vi "ConvertTextBasedCodeToLabVIEW_AttToHtml.vi"(7 "MissingClasses":string[](array[string]), 10 "ShowAccesScope(True)":bool=TRUE, 11 "DataType":T1) -> (3 "String":string)   [LabVIEW 2020]
uses:
  <resource>/Framework/Providers/Open_GDS/ClassProviders/Common/CommonVIs/CommonVIs_AttributeType.ctl
  <resource>/Framework/Providers/Open_GDS/ClassProviders/Common/CommonVIs/CommonVIs_AttributeDataType.ctl
  <resource>/Framework/Providers/Open_GDS/ClassProviders/Common/String/GDSString_AccessScopeModifierType.ctl
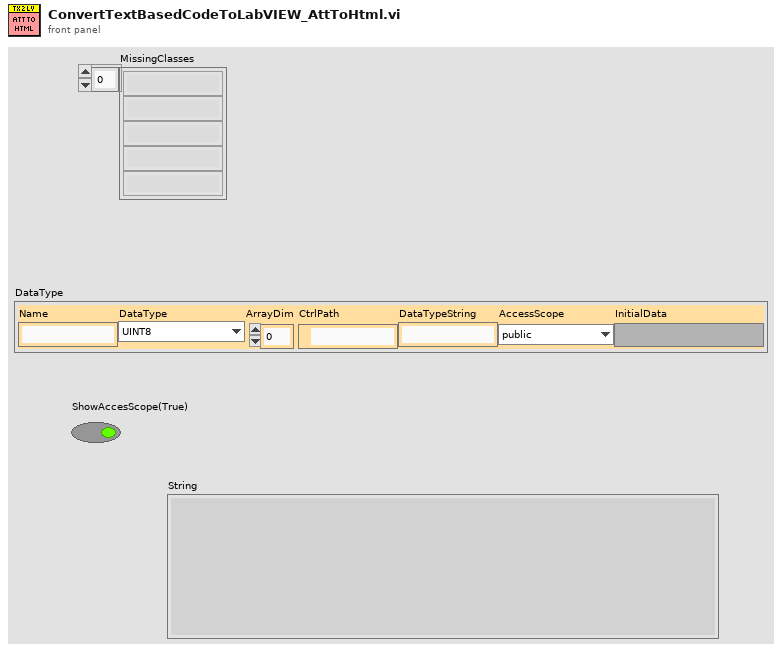
[diagram p1: front panel]
types:
  T1 = typedef "CommonVIs_AttributeType.ctl" = cluster{"Name":string, "DataType":T2, "ArrayDim":i32, "CtrlPath":path, "DataTypeString":string, "AccessScope":T3, "InitialData":variant}
  T2 = typedef "CommonVIs_AttributeDataType.ctl" = enum16{"UINT8", "INT8", "UINT16", "INT16", "UINT32", "INT32", "UINT64", "INT64", "SGL", "DBL", "EXT", "CSG", "CDB", "CXT", "TimeStamp", "STRING", "PATH", "BOOL", "ENUM", "RefNum", "VIRefNum", "LabVIEW Class", "Cluster", "Variant", "TypeDef", "Waveform", "LabVIEW Object", "Other", "void"}
  T3 = typedef "GDSString_AccessScopeModifierType.ctl" = enum16{"public", "private", "protected", "internal"}
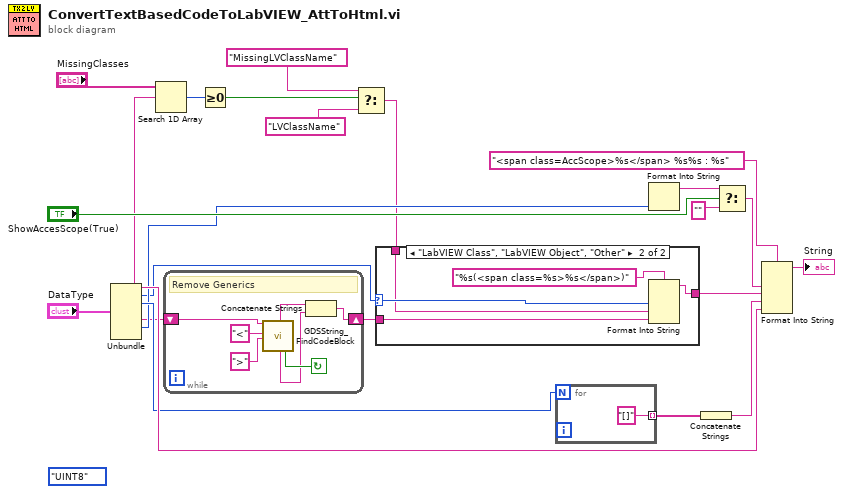
[diagram p0: block diagram]
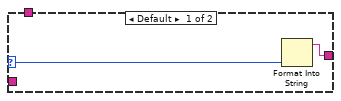
[diagram p2: hidden frame]
diagram:
  (unwired) CommonVIs_AttributeDataType."UINT8" ("DataType")
  n1 = Unbundle("DataType") -> ("Name"=w22:string, "DataType"=w9:T2, "ArrayDim"=w19:i32, "DataTypeString"=w6:string, "AccessScope"=w12:T3)  [unwired: 2 out]
  n2 = Search 1D Array(1D array="MissingClasses", element=w6) -> (index of element=w5:i32)  [unwired: 1 in]
  n3 = while {
    shift-right: [w23] -> w8
    shift-left: w6 -> [w29]
    stop <- w26 continue-if-true
    # "Remove Generics"
    n4 = call <resource>:"GDSString_FindCodeBlock.vi"("Text"=w29, "CodeBlockStartCharacter( { )"="<", "CodeBlockEndCharacter( } )"=">") -> ("TextBeforeBlock"=w25:string, "TextAfterBlock"=w24:string, "found"=w26:bool)  [unwired: 8 in, 6 out]
    n5 = Concatenate Strings(w25, w24) -> (w23:string)
  }
  n6 = Greater Or Equal To 0?(x=w5) -> (x >= 0?=w4:bool)
  n7 = Select(t="MissingLVClassName" ("CodeBlockStartCharacter( { )"), s=w4, f="LVClassName" ("CodeBlockStartCharacter( { )")) -> (s? t:f=w1:string)
  n8 = case shown="\"LabVIEW Class\", \"LabVIEW Object\", \"Other\"" w9 {
    selector: w9 -> [w31 w33]
    tunnel: [w30 w35] -> w10
    tunnel: w8 -> [_ w34]
    tunnel: w1 -> [_ w32]
    frame Default {
      n9 = Format Into String(w31) -> (resulting string=w30:string)  [unwired: 3 in, 1 out]
    }
    frame "LabVIEW Class", "LabVIEW Object", "Other" {
      n10 = Format Into String(format string="%s(<span class=%s>%s</span>)", w33, w32, w34) -> (resulting string=w35:string)  [unwired: 2 in, 1 out]
    }
  }
  n11 = for {
    N: w19 -> [_]
    tunnel: ["[]"] -> w20 mode=indexing
  }
  n12 = Format Into String(w12) -> (resulting string=w14:string)  [unwired: 3 in, 1 out]
  n13 = Concatenate Strings(w20) -> (w21:string)
  n14 = Select(t=w14, s="ShowAccesScope(True)", f="") -> (s? t:f=w11:string)
  n15 = Format Into String(format string="<span class=AccScope>%s</span> %s%s : %s", w11, w10, w21, w22) -> (resulting string=→"String":string)  [unwired: 2 in, 1 out]
